vi "Close_Baxter.vi"(0 "error in":errorcluster, 2 "topic":string) -> (1 "error out":errorcluster)   [LabVIEW 2010]
doc: "Closes a topic. If no topic is defined, it will close all tasks and close the console (unless specified otherwise)."
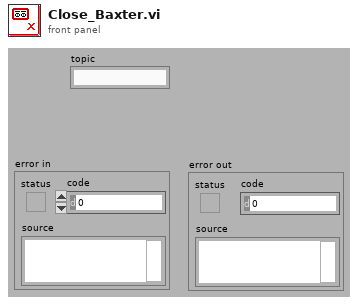
[diagram p1: front panel]
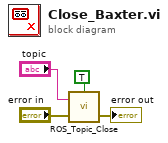
[diagram p0: block diagram]
diagram:
  n1 = call "ROS_Topic_Close.vi"("error in"="error in", "topic"="topic", "StopConsole"=TRUE) -> ("error out"=→"error out":errorcluster)  [unwired: 1 in]
